vi "Stepped Frequency Sweep.vi"(0 "Semiconductor Module Context":T2, 1 "Coarse Frequency Sweep (Hz)":T1={"Start"=20.0, "End"=20000.0, "Samples"=128} {"End" format="%#_13g"; "Start" format="%#_13g"}, 2 "Fine Frequency Sweep (Hz)":T1={"Start"=20.0, "End"=20000.0, "Samples"=128} {"End" format="%#_13g"; "Start" format="%#_13g"}, 5 "Speaker Sampling Rate (Hz)":dbl=1100.0 format="%#_13g", 7 "Ref Mic Sampling Rate (Hz)":dbl=1100.0 format="%#_13g", 9 "Amplitude (V)":dbl=0.01 format="%#_13g", 11 "error in (no error)":errorcluster) -> (4 "Frequency (Hz)":dbl[](array[numeric]), 6 "Per-Site Per-Frequency dbSPL":dbl[][](array[numeric]), 15 "error out":errorcluster)   [LabVIEW 2020]
doc: "Stepped Frequency Sweep is used to perform a Frequency sweep for a constant amplitude voltage under a given sampling rate to obtain the equivalent Per-Site dB SPL"
uses:
  <vilib>/NI_TestStand_SemiconductorModule/NI_TestStand_Semiconductor_Module.lvlibp/PinMap/General/SemiconductorModuleContext.ctl
  Common/Utility/Calibration Sweep/Sweep Parameters.ctl
  e4dca00a-4e93-4fe6-a22a-85184fe6c6d7.vi
  6f0c4c81-6e94-4ac5-a946-327ae8ed193a.vi
  3fa66fd1-3a97-4e0c-9204-a9f8b558bf39.vi
  <vilib>/measure/matone.llb/Extract Single Tone Information N Chan.vi
  <vilib>/NI_TestStand_SemiconductorModule/NI_TestStand_Semiconductor_Module.lvlibp
  <vilib>/measure/NI_MAPro.lvlib
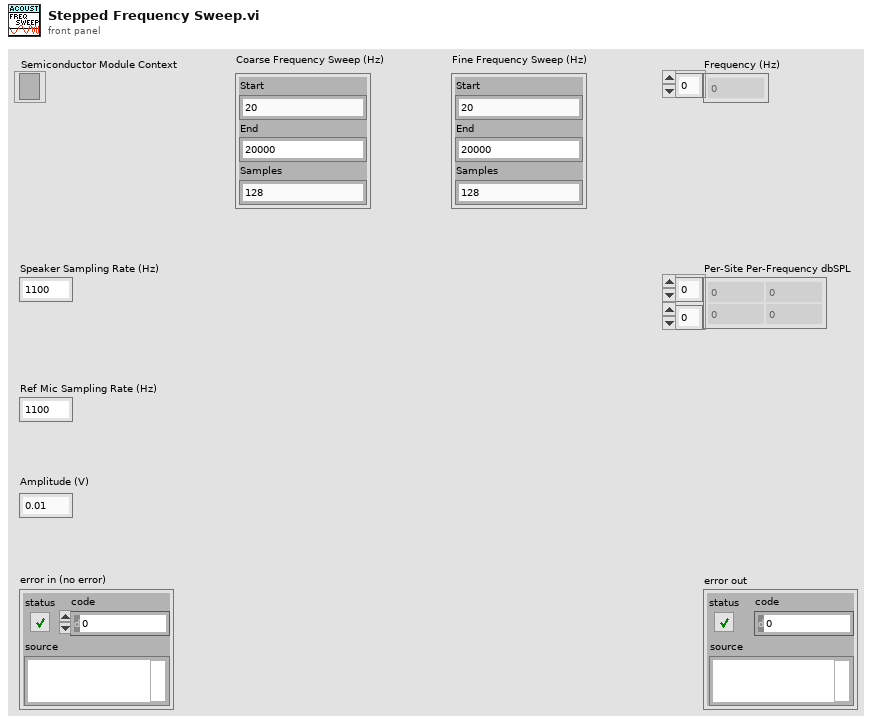
[diagram p1: front panel]
types:
  T1 = typedef "Sweep Parameters.ctl" = cluster{"Start":dbl, "End":dbl, "Samples":i32}
  T2 = typedef "NI_TestStand_Semiconductor_Module.lvlibp/SemiconductorModuleContext.ctl" = refnum<k7>
  T3 = typedef "TSM DAQmx Multi-Task.ctl" = cluster{"Pin Query Context":refnum<class "MultiplePinMultipleSessionQueryContext.lvclass">, "SSC":T4[], "Site Numbers":i32[], "Pins":tag[]}
  T4 = typedef "SSC DAQmx.ctl" = cluster{"DAQmx Task ":refnum<k21>, "Channels":string, "Channel Lists":string}
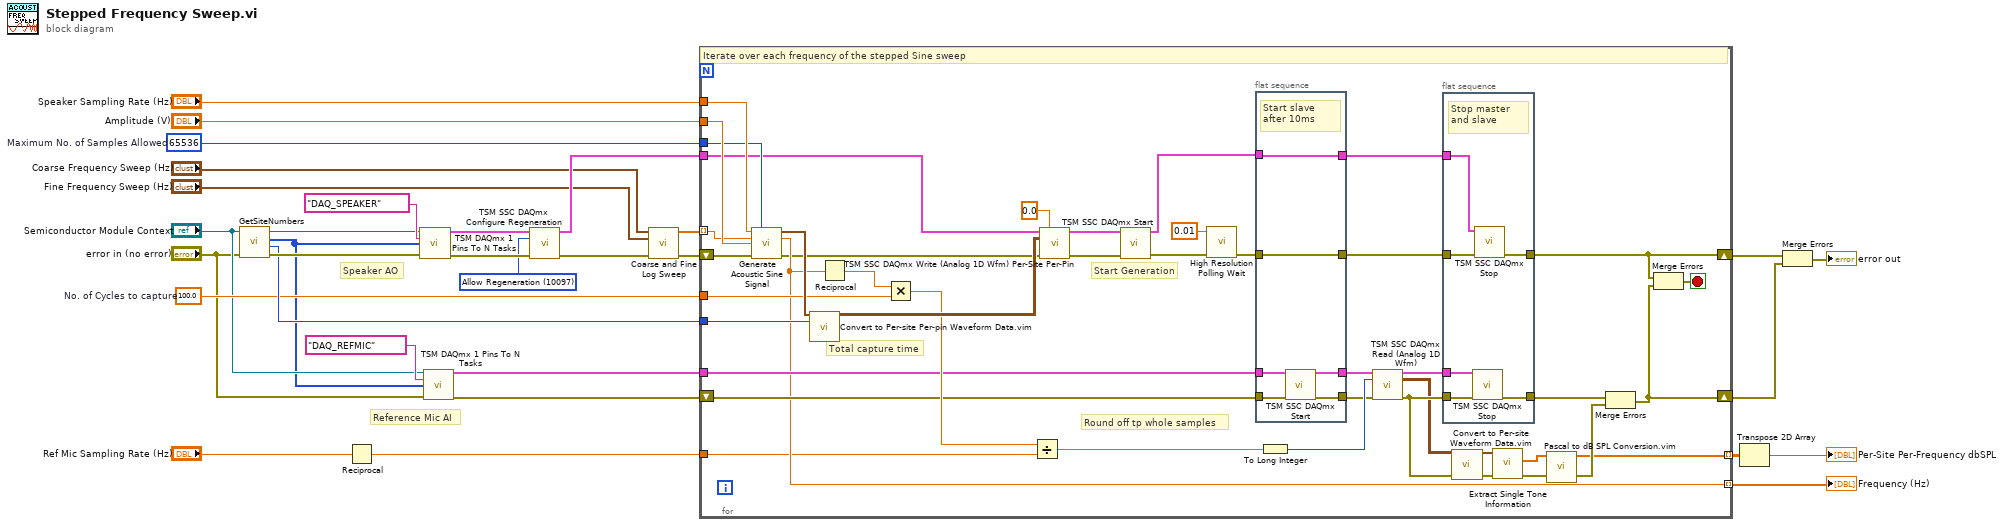
[diagram p0: block diagram]
diagram:
  w1 = 10097 items=["Allow Regeneration"=10097, "Do Not Allow Regeneration"=10158] ("RegenMode")
  w17 = 65536  # Maximum No. of Samples Allowed
  w20 = 100.0  # No. of Cycles to capture
  # "Reference Mic AI"
  # "Speaker AO"
  n1 = call <vilib>:"GetSiteNumbers.vi"("error in (no error)"="error in (no error)", "Semiconductor Module Context"="Semiconductor Module Context") -> ("error out"=w27:errorcluster, "Number Of Sites"=w21:i32, "Site Numbers"=w6:i32[], "Semiconductor Module Context Out"=w28:T2)  [unwired: 6 in]
  n2 = Reciprocal(x="Ref Mic Sampling Rate (Hz)") -> (1/x=w2:dbl)
  n3 = call "TSM DAQmx 1 Pins To N Tasks.vi"("TSM context"=w28, "Pins"=tag "DAQ_SPEAKER", "Site Numbers"=w6, "error in"=w27) -> ("DAQ TSM Out"=w30:T3, "error out"=w31:errorcluster)  [unwired: 10 in]
  n4 = call "TSM DAQmx 1 Pins To N Tasks.vi"("TSM context"="Semiconductor Module Context", "Pins"=tag "DAQ_REFMIC", "Site Numbers"=w6, "error in"="error in (no error)") -> ("DAQ TSM Out"=w13:T3, "error out"=w14:errorcluster)  [unwired: 10 in]
  n5 = call "TSM SSC DAQmx Configure Regeneration.vi"("TSM DAQmx In"=w30, "RegenMode"=w1, "error in (no error)"=w31) -> ("TSM DAQmx Out"=w26:T3, "error out"=w11:errorcluster)  [unwired: 11 in]
  n6 = call "Coarse and Fine Log Sweep.vi"("Coarse Sweep"="Coarse Frequency Sweep (Hz)", "Fine Sweep"="Fine Frequency Sweep (Hz)", "error in (no error)"=w11) -> ("Sweep Values"=w10:dbl[], "error out"=w25:errorcluster)  [unwired: 11 in]
  n7 = for {
    shift-right: [w41] -> w19
    shift-left: w25 -> [w72]
    tunnel: w10 -> [w70] mode=indexing
    shift-right: [w40] -> w15
    shift-left: w14 -> [w53]
    tunnel: "Amplitude (V)" -> [w71]
    tunnel: "Speaker Sampling Rate (Hz)" -> [w59]
    tunnel: w21 -> [w61]
    tunnel: w20 -> [w67]
    tunnel: w17 -> [w55]
    tunnel: w13 -> [w52]
    tunnel: w26 -> [w32]
    tunnel: [w37] -> w8 mode=indexing
    tunnel: [w36] -> w9 mode=indexing
    tunnel: w2 -> [w34]
    stop <- w39 stop-if-true
    # "Start Generation"
    # "Round off tp whole samples"
    # "Total capture time"
    # "Iterate over each frequency of the stepped Sine sweep"
    n8 = call "Generate Acoustic Sine Signal.vi"("Sampling Rate"=w59, "Maximum No. of Samples Allowed"=w55, "Frequency"=w70, "Sine wave amplitude"=w71, "error in (no error)"=w72) -> ("waveform"=w68:waveform(dbl), "Actual Frequency"=w37:dbl, "error out"=w33:errorcluster)  [unwired: 8 in]
    n9 = call "Convert to Per-site Per-pin Waveform Data.vim"("Waveform In"=w68, "No. of Site"=w61) -> ("Per Site Per Pin Waveform Out"=w69:waveform(dbl)[][])  [unwired: 13 in]
    n10 = Reciprocal(x=w37) -> (1/x=w45:dbl)
    n11 = Multiply(x=w45, y=w67) -> (x*y=w58:dbl)
    n12 = Divide(x=w58, y=w34) -> (x/y=w57:dbl)
    n13 = call "TSM SSC DAQmx Write (Analog 1D Wfm) Per-Site Per-Pin.vi"("DAQ TSM in"=w32, "Idle Channel Value (0)"=0.0, "Per-Site Per-Pin Waveforms in"=w69, "error in"=w33) -> ("DAQ TSM Out"=w66:T3, "error out"=w63:errorcluster)  [unwired: 10 in]
    n14 = call "TSM SSC DAQmx Start.vi"("TSM DAQmx In"=w66, "error in (no error)"=w63) -> ("TSM DAQmx Out"=w49:T3, "error out"=w60:errorcluster)  [unwired: 12 in]
    n15 = call <vilib>:"High Resolution Polling Wait.vi"("error in (no error)"=w60, "seconds to wait"=0.01) -> ("error out"=w47:errorcluster)  [unwired: 9 in]
    n16 = flat-sequence {
      tunnel: w53 -> [w78]
      tunnel: w52 -> [w77]
      tunnel: [w76] -> w51
      tunnel: [w75] -> w50
      tunnel: w49 -> [w74]
      tunnel: [w74] -> w48
      tunnel: w47 -> [w73]
      tunnel: [w73] -> w46
      frame #0 {
        # "Start slave after 10ms"
        n17 = call "TSM SSC DAQmx Start.vi"("TSM DAQmx In"=w77, "error in (no error)"=w78) -> ("TSM DAQmx Out"=w75:T3, "error out"=w76:errorcluster)  [unwired: 12 in]
      }
    }
    n18 = To Long Integer(number=w57) -> (32bit integer=w56:i32)
    n19 = call "TSM SSC DAQmx Read (Analog 1D Wfm).vi"("DAQ TSM in"=w50, "Samples to read"=w56, "error in"=w51) -> ("DAQ TSM Out"=w65:T3, "Per-Site Per-Pin Waveforms Out"=w38:waveform(dbl)[][], "error out"=w44:errorcluster)  [unwired: 10 in]
    n20 = flat-sequence {
      tunnel: w46 -> [w84]
      tunnel: w48 -> [w83]
      tunnel: [w82] -> w41
      tunnel: w44 -> [w81]
      tunnel: [w80] -> w43
      tunnel: w65 -> [w79]
      frame #0 {
        # "Stop master and slave"
        n21 = call "TSM SSC DAQmx Stop.vi"("TSM DAQmx In"=w79, "error in (no error)"=w81) -> ("error out"=w80:errorcluster)  [unwired: 12 in, 1 out]
        n22 = call "TSM SSC DAQmx Stop.vi"("TSM DAQmx In"=w83, "error in (no error)"=w84) -> ("error out"=w82:errorcluster)  [unwired: 12 in, 1 out]
      }
    }
    n23 = call "Convert to Per-site Waveform Data.vim"("Per-Site Per-Pin Waveform In"=w38) -> ("Per-Site Waveform Out"=w64:waveform(dbl)[])  [unwired: 14 in]
    n24 = call-poly <vilib>:"Extract Single Tone Information.vi"("error in (no error)"=w44, "time signals in"=w64) -> ("error out"=w42:errorcluster, "detected amplitudes"=w35:dbl[])  [unwired: 4 in, 4 out]
    n25 = call "Pascal to dB SPL Conversion.vim"("Pascals"=w35) -> ("dbSPL"=w36:dbl[])  [unwired: 14 in]
    n26 = Merge Errors(w43, w42) -> (w40:errorcluster)
    n27 = Merge Errors(w41, w40) -> (w39:errorcluster)
  }
  "Frequency (Hz)" <- w8
  n28 = Transpose 2D Array(2D array=w9) -> (transposed array=→"Per-Site Per-Frequency dbSPL":dbl[][])
  n29 = Merge Errors(w19, w15) -> (→"error out":errorcluster)
